vi "TA_Generate_DelayTime_Linear.vi"(10 "Step (ps)":dbl[](array[numeric])=[0.5, 0.05, 0.1, 0.5, 1.0, 2.0, 10.0, 100.0], 11 "Time Range (ps)":dbl[](array[numeric])=[-10.0, -1.0, 1.0, 5.0, 20.0, 100.0, 500.0, 1000.0, 8000.0]) -> (2 "Number (Delay Time)":i32, 3 "Generated Delay Time (ps)":dbl[](array[numeric]))   [LabVIEW 2025]
uses:
  <vilib>/Analysis/1siggen.llb/Ramp Pattern by Delta.vi
  <vilib>/Analysis/NI_AALBase.lvlib
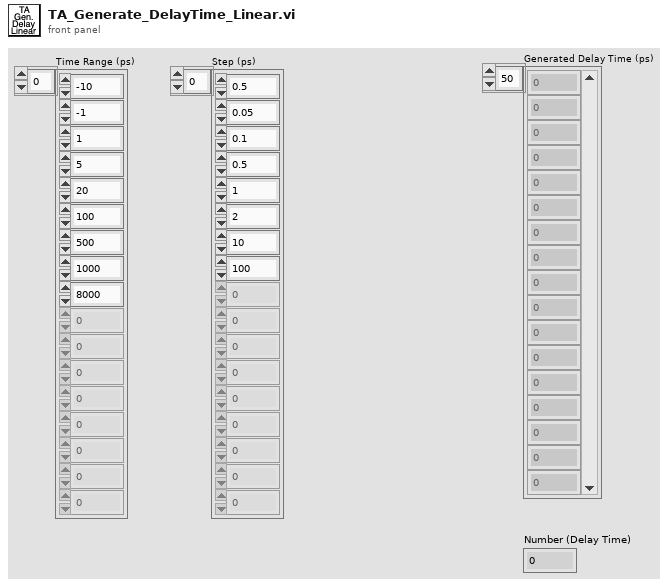
[diagram p1: front panel]
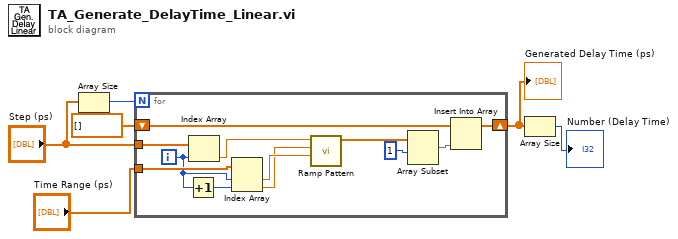
[diagram p0: block diagram]
diagram:
  n1 = Array Size(array="Step (ps)") -> (size(s)=w5:i32)
  n2 = for {
    N: w5 -> [_]
    tunnel: "Time Range (ps)" -> [w18]
    tunnel: "Step (ps)" -> [w14]
    shift-right: [w10] -> w2
    shift-left: dbl[] [] ("Array") -> [w11]
    i -> [w12]
    n3 = Increment(x=w12) -> (x+1=w17:i32)
    n4 = Index Array(array=w14, index=w12) -> (element=w13:dbl)
    n5 = Index Array(array=w18, index #1=w12, index #2=w17) -> (element #1=w16:dbl, element #2=w15:dbl)
    n6 = call-poly <vilib>:"Ramp Pattern.vi"("start"=w16, "end"=w15, "delta"=w13) -> ("Ramp Pattern"=w9:dbl[])  [unwired: 6 in, 2 out]
    n7 = Array Subset(array=w9, index=1) -> (w7:dbl[])  [unwired: 1 in]
    n8 = Insert Into Array(array=w11, new element=w7) -> (w10:dbl[])  [unwired: 1 in]
  }
  "Generated Delay Time (ps)" <- w2
  n9 = Array Size(array=w2) -> (size(s)=→"Number (Delay Time)":i32)
